vi "Launch New Chat Window.vi"(8 "error in (no error)":errorcluster, 11 "Server in":refnum<class "Server.lvclass">) -> (0 "error out":errorcluster, 3 "Server out":refnum<class "Server.lvclass">)   [LabVIEW 2015, in "Server.lvlib" / "Server.lvclass"]
uses:
  Server.lvclass
  <vilib>/ActorFramework/Actor/Actor.lvclass
  Chat Window Model/Chat Window Model/Chat Window Model.lvclass
  Server Messages/Status Update Msg/Status Update Msg.lvclass
  Server Messages/Direct Message Recieved Msg/Direct Message Recieved Msg.lvclass
  Chat Window Model/Chat Window Model Messages/Update Online List Msg/Update Online List Msg.lvclass
  Chat Window Model/Chat Window Model Messages/Update Status Log Msg/Update Status Log Msg.lvclass
  Server Messages/Enable Controls Msg/Enable Controls Msg.lvclass
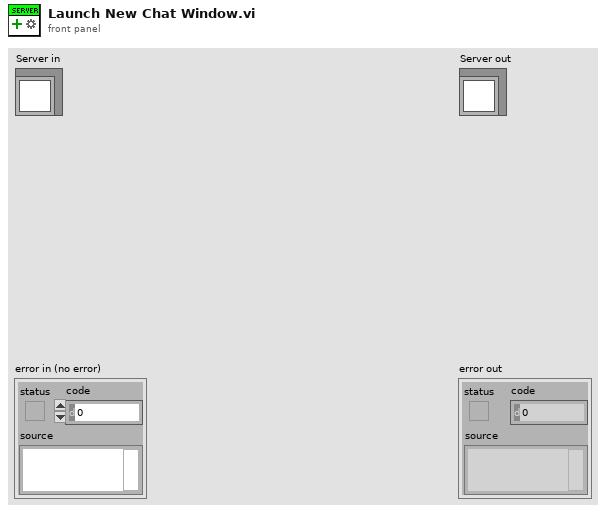
[diagram p1: front panel]
types:
  T1 = enum8{"Enabled", "Disabled", "Disabled and Grayed Out"}
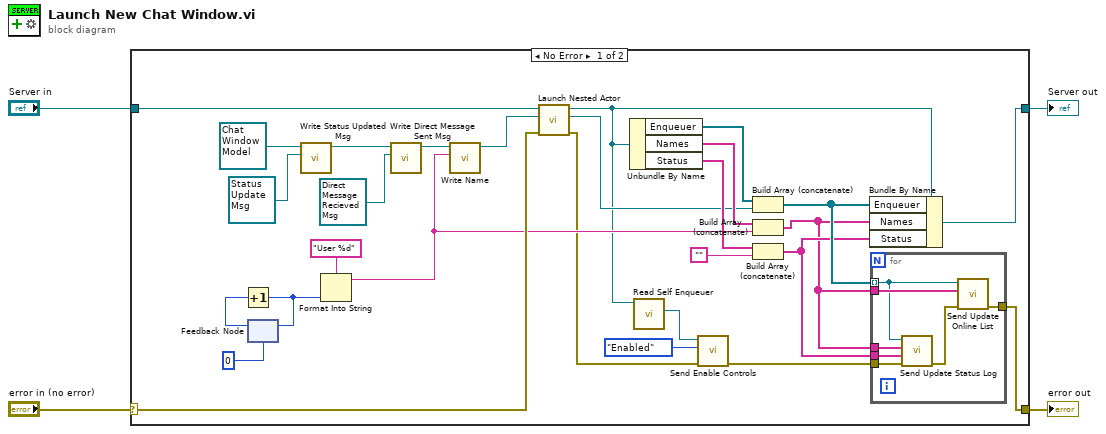
[diagram p0: block diagram]
diagram:
  n1 = case shown="No Error" "error in (no error)" {
    selector: "error in (no error)" -> [w31 w41]
    tunnel: [w10 w41] -> w3
    tunnel: [w14 w40] -> w1
    tunnel: "Server in" -> [w32 w40]
    frame No Error {
      n2 = feedback #1(0) -> (w28:i32)
      n3 = Increment(x=w28) -> (x+1=w26:i32)
      n4 = feedback-in #1(w26) -> ()
      n5 = call "Write Status Updated Msg.vi"("Chat Window Model.lvlib:Status Updated Msg.lvclass"=refnum<class "Status Update Msg.lvclass"> refnum ("Server.lvlib:Status Update Msg.lvclass"), "Chat Window Model in"=refnum<class "Chat Window Model.lvclass"> refnum ("Chat Window Model.lvlib:Chat Window Model.lvclass")) -> ("Chat Window Model out"=w23:refnum<class "Chat Window Model.lvclass">)  [unwired: 9 in]
      n6 = Format Into String(format string="User %d", w26) -> (resulting string=w16:string)  [unwired: 2 in, 1 out]
      n7 = call "Write Direct Message Sent Msg.vi"("Chat Window Model.lvlib:Direct Message Sent Msg.lvclass"=refnum<class "Direct Message Recieved Msg.lvclass"> refnum ("Server.lvlib:Direct Message Recieved Msg.lvclass"), "Chat Window Model in"=w23) -> ("Chat Window Model out"=w22:refnum<class "Chat Window Model.lvclass">)  [unwired: 9 in]
      n8 = call "Write Name.vi"("Name"=w16, "Chat Window Model in"=w22) -> ("Chat Window Model out"=w30:refnum<class "Chat Window Model.lvclass">)  [unwired: 8 in, 1 out]
      n9 = call <vilib>:"Launch Nested Actor.vi"("error in (no error)"=w31, "Nested Actor"=w30, "Caller Actor in"=w32) -> ("error out"=w8:errorcluster, "Nested Actor's Enqueuer"=w17:refnum<class "Message Enqueuer.lvclass">, "Caller Actor out"=w7:refnum<class "Server.lvclass">)  [unwired: 6 in]
      n10 = Unbundle By Name(w7) -> ("Enqueuer"=w20:refnum<class "Message Enqueuer.lvclass">[], "Names"=w19:string[], "Status"=w18:string[])
      n11 = call <vilib>:"Read Self Enqueuer.vi"("Actor"=w7) -> ("Self Enqueuer"=w6:refnum<class "Message Enqueuer.lvclass">)  [unwired: 10 in]
      n12 = call "Send Enable Controls.vi"("error in (no error)"=w8, "Disabled"=T1."Enabled", "Message Enqueuer"=w6) -> ("error out"=w9:errorcluster)  [unwired: 7 in, 1 out]
      n13 = Build Array (concatenate)(w20, w17) -> (w13:refnum<class "Message Enqueuer.lvclass">[])
      n14 = Build Array (concatenate)(w19, w16) -> (w11:string[])
      n15 = Build Array (concatenate)(w18, "") -> (w12:string[])
      n16 = Bundle By Name(cluster=w7, "Enqueuer"=w13, "Names"=w11, "Status"=w12) -> (w14:refnum<class "Server.lvclass">)
      n17 = for {
        tunnel: w13 -> [w38] mode=indexing
        tunnel: w11 -> [w39]
        tunnel: w12 -> [w37]
        tunnel: w11 -> [w36]
        tunnel: [w34] -> w10
        tunnel: w9 -> [w33]
        n18 = call "Send Update Status Log.vi"("error in (no error)"=w33, "Status List"=w37, "Names"=w36, "Message Enqueuer"=w38) -> ("error out"=w35:errorcluster)  [unwired: 6 in, 1 out]
        n19 = call "Send Update Online List.vi"("error in (no error)"=w35, "Online Users"=w39, "Message Enqueuer"=w38) -> ("error out"=w34:errorcluster)  [unwired: 7 in, 1 out]
      }
    }
    frame Error {
    }
  }
  "error out" <- w3
  "Server out" <- w1
